vi "unescape string perf.vi"() -> ()   [LabVIEW 2017]
uses:
  JSONtext.lvlib
panel:
  in  "max length before escape":i32=10000000
  out "length after":i32
  out "length before":i32
  out "ds=":bool[](array[boolean])
  in  "unicode":bool=TRUE
  out "Array 2":string[](array[string])
  out "t":dbl[](array[numeric])=[1.4827295089180552, 2.8257225429488244, 2.876002117587632]
  # "lvjson"
  # "ds"
  # "lvjson"
  # "jsontxt"
  # "jsontxt"
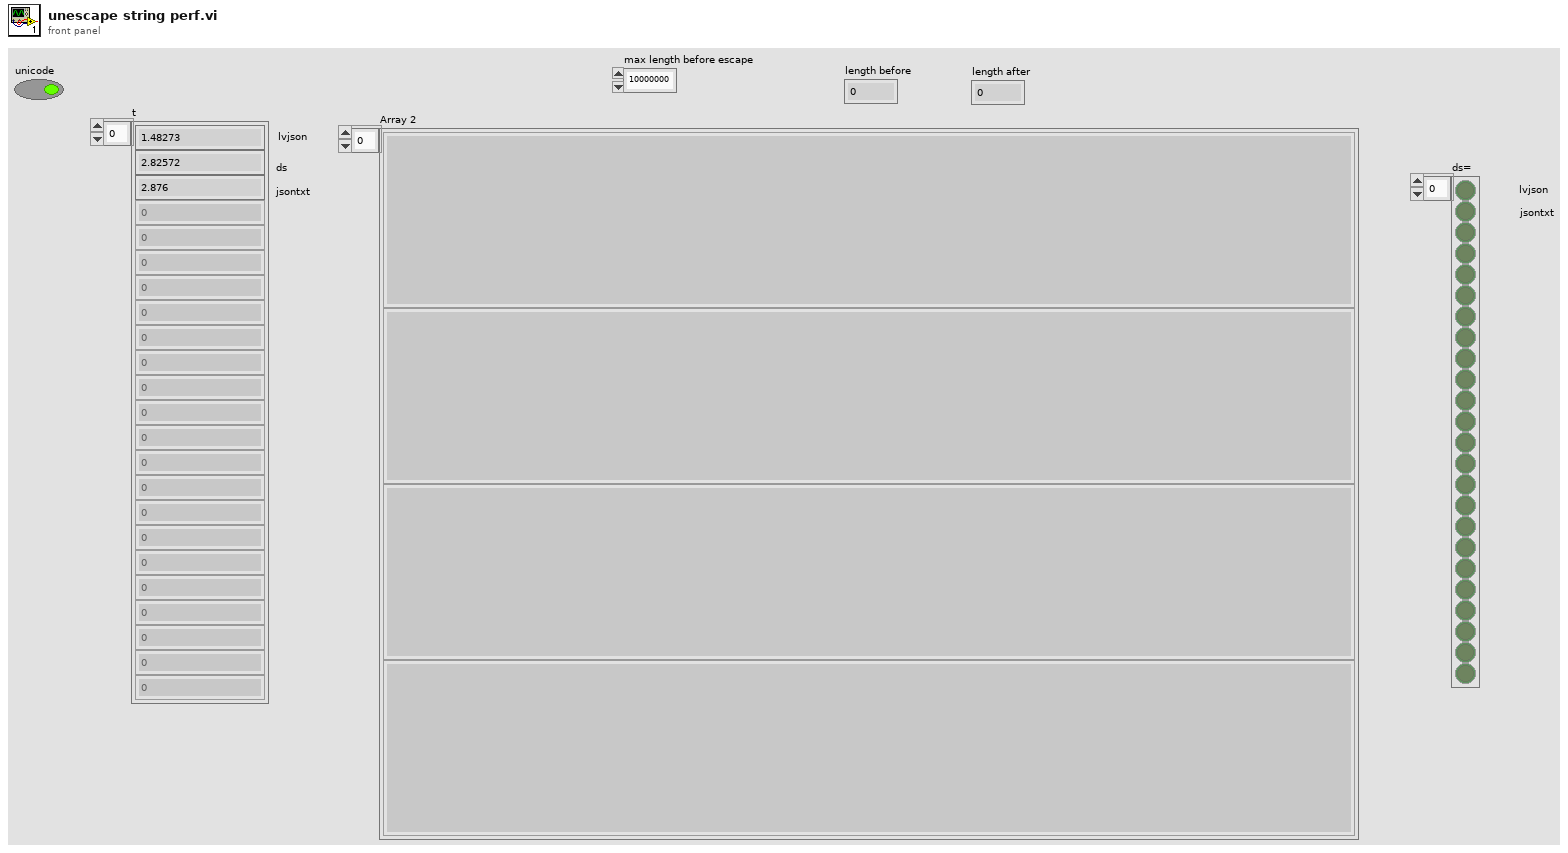
[diagram p1: front panel]
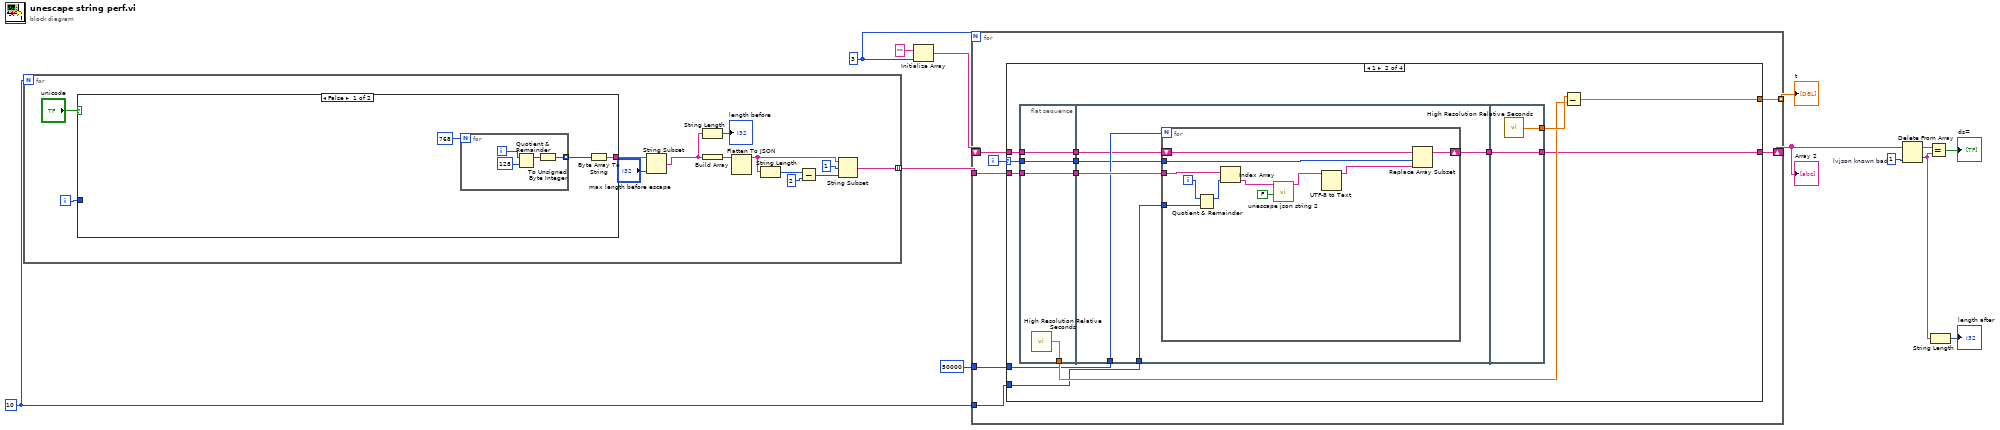
[diagram p0: block diagram]
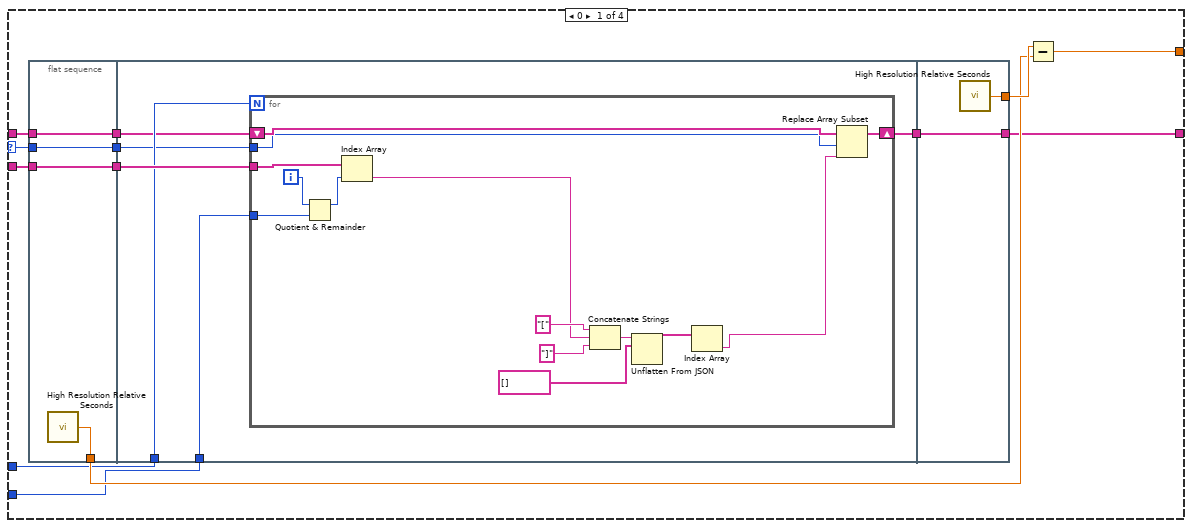
[diagram p2: hidden frame]
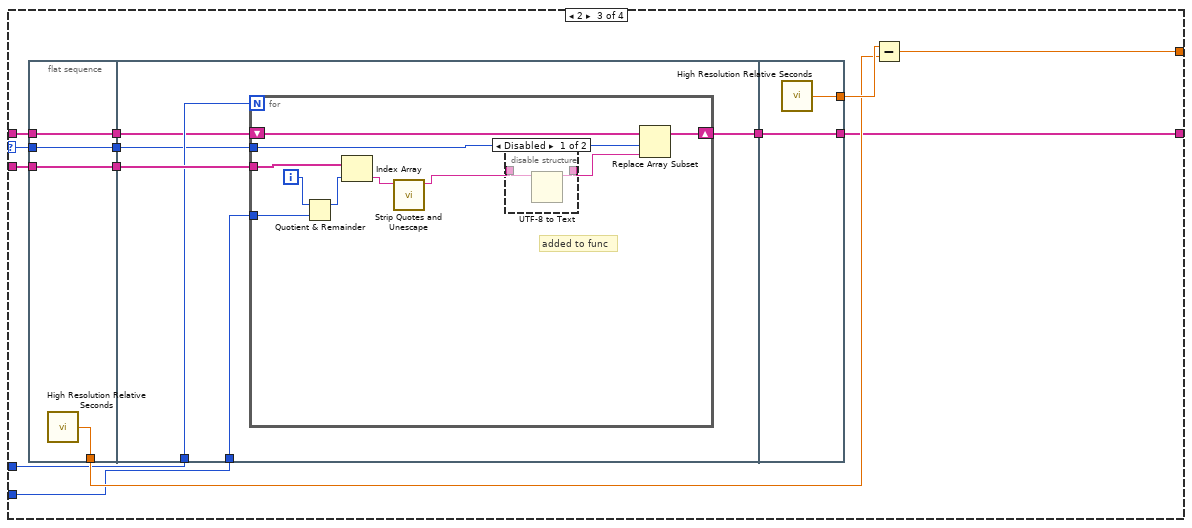
[diagram p3: hidden frame]
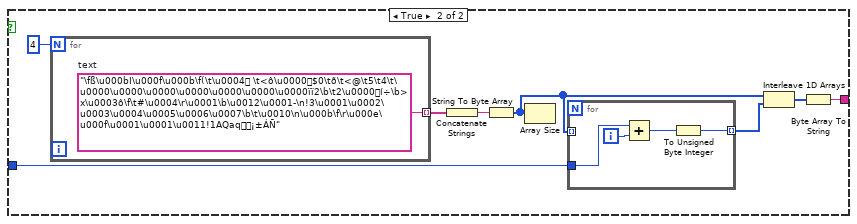
[diagram p6: hidden frame]
diagram:
  w4 = 1  # lvjson known bad
  w8 = 3
  w12 = 10
  n1 = for {
    N: w12 -> [_]
    tunnel: [w16] -> w10 mode=indexing
    i -> [w26]
    n2 = case shown="False" "unicode" {
      tunnel: w26 -> [_ w40]
      tunnel: [w27 w36] -> w17
      frame False {
        n3 = for {
          N: 768 -> [_]
          tunnel: [w30] -> w28 mode=indexing
          i -> [w33]
          n4 = Quotient & Remainder(x=w33, y=128) -> (x-y*floor(x/y)=w31:i32)  [unwired: 1 out]
          n5 = To Unsigned Byte Integer(number=w31) -> (unsigned 8bit integer=w30:u8)
        }
        n6 = Byte Array To String(unsigned byte array=w28) -> (string=w27:string)
      }
      frame True {
        n7 = for {
          N: 4 -> [_]
          tunnel: [w42] -> w41 mode=indexing
          w42 = "\fß\u000bI\u000f\u000b\f(\t\u0004 \t<ô\u0000$0\tð\t<@\t5\t4\t\u0000\u0000\u0000\u0000\u0000\u0000\u0000ïï2\b\t2\u0000í÷\b> x\u0003ô\f\t#\u0004\r\u0001\b\u0012\u0001-\n!3\u0001\u0002\u0003\u0004\u0005\u0006\u0007\b\t\u0010\n\u000b\f\r\u000e\u000f\u0001\u0001\u0011!1AQaq¡±ÁÑ"  # text
        }
        n8 = Concatenate Strings(w41) -> (w34:string)
        n9 = String To Byte Array(string=w34) -> (unsigned byte array=w38:u8[])
        n10 = Array Size(array=w38) -> ()  [unwired: 1 out]
        n11 = for {
          tunnel: w38 -> [_] mode=indexing
          tunnel: w40 -> [w45]
          tunnel: [w43] -> w39 mode=indexing
          i -> [w46]
          n12 = Add(x=w45, y=w46) -> (x+y=w44:i32)
          n13 = To Unsigned Byte Integer(number=w44) -> (unsigned 8bit integer=w43:u8)
        }
        n14 = Interleave 1D Arrays(w38, w39) -> (w37:u8[])
        n15 = Byte Array To String(unsigned byte array=w37) -> (string=w36:string)
      }
    }
    n16 = String Subset(string=w17, length (rest)="max length before escape") -> (substring=w15:string)  [unwired: 1 in]
    n17 = String Length(string=w15) -> (length=→"length before":i32)
    n18 = Build Array(w15) -> (w23:string[])
    n19 = Flatten To JSON(anything=w23) -> (JSON string=w21:string)  [unwired: 2 in, 1 out]
    n20 = String Length(string=w21) -> (length=w20:i32)
    n21 = Subtract(x=w20, y=2) -> (x-y=w18:i32)
    n22 = String Subset(string=w21, offset (0)=1, length (rest)=w18) -> (substring=w16:string)
  }
  n23 = Initialize Array("", w8) -> (w7:string[])
  n24 = for {
    N: w8 -> [_]
    tunnel: w10 -> [w51]
    tunnel: [w52] -> w13 mode=indexing
    tunnel: w12 -> [w50]
    tunnel: 50000 -> [w49]
    shift-right: [w47] -> w6
    shift-left: w7 -> [w48]
    i -> [w53]
    n25 = case shown="1" w53 {
      selector: w53 -> [w55 w94 w130 _]
      tunnel: [w64 w103 w139 _] -> w52
      tunnel: w51 -> [w62 w101 w137 _]
      tunnel: w50 -> [w61 w100 w136 _]
      tunnel: w49 -> [w60 w99 w135 _]
      tunnel: w48 -> [w59 w98 w134 w167]
      tunnel: [w57 w96 w132 w167] -> w47
      frame 0 {
        n26 = flat-sequence {
          tunnel: [w70] -> w65
          tunnel: [w69] -> w63
          tunnel: w62 -> [w69]
          tunnel: w59 -> [w68]
          tunnel: [w68] -> w58
          tunnel: w55 -> [w67]
          tunnel: [w67] -> w54
          tunnel: w63 -> [w75]
          tunnel: w61 -> [w76]
          tunnel: w60 -> [w74]
          tunnel: w58 -> [w73]
          tunnel: [w72] -> w56
          tunnel: w54 -> [w71]
          tunnel: [w92] -> w66
          tunnel: [w91] -> w57
          tunnel: w56 -> [w91]
          frame #0 {
            n27 = call <vilib>:"High Resolution Relative Seconds.vi"() -> ("relative seconds"=w70:dbl)
          }
          frame #1 {
            n28 = for {
              N: w74 -> [_]
              tunnel: w76 -> [w89]
              tunnel: w75 -> [w87]
              shift-right: [w85] -> w72
              shift-left: w73 -> [w86]
              tunnel: w71 -> [w84]
              i -> [w90]
              n29 = Quotient & Remainder(x=w90, y=w89) -> (x-y*floor(x/y)=w88:i32)  [unwired: 1 out]
              n30 = Index Array(array=w87, index=w88) -> (element=w78:string)
              n31 = Concatenate Strings("[", w78, "]") -> (w80:string)
              n32 = Unflatten From JSON(JSON string=w80, type and defaults=string[] []) -> (value=w79:string[])  [unwired: 5 in, 1 out]
              n33 = Index Array(array=w79) -> (element=w77:string)  [unwired: 1 in]
              n34 = Replace Array Subset(array=w86, new element=w77, index=w84) -> (w85:string[])
            }
          }
          frame #2 {
            n35 = call <vilib>:"High Resolution Relative Seconds.vi"() -> ("relative seconds"=w92:dbl)
          }
        }
        n36 = Subtract(x=w66, y=w65) -> (x-y=w64:dbl)
      }
      frame 1 {
        n37 = flat-sequence {
          tunnel: [w109] -> w104
          tunnel: [w108] -> w102
          tunnel: w101 -> [w108]
          tunnel: w98 -> [w107]
          tunnel: [w107] -> w97
          tunnel: w94 -> [w106]
          tunnel: [w106] -> w93
          tunnel: w102 -> [w114]
          tunnel: w100 -> [w115]
          tunnel: w99 -> [w113]
          tunnel: w97 -> [w112]
          tunnel: [w111] -> w95
          tunnel: w93 -> [w110]
          tunnel: [w128] -> w105
          tunnel: [w127] -> w96
          tunnel: w95 -> [w127]
          frame #0 {
            n38 = call <vilib>:"High Resolution Relative Seconds.vi"() -> ("relative seconds"=w109:dbl)
          }
          frame #1 {
            n39 = for {
              N: w113 -> [_]
              tunnel: w115 -> [w125]
              tunnel: w114 -> [w123]
              shift-right: [w121] -> w111
              shift-left: w112 -> [w122]
              tunnel: w110 -> [w120]
              i -> [w126]
              n40 = Quotient & Remainder(x=w126, y=w125) -> (x-y*floor(x/y)=w124:i32)  [unwired: 1 out]
              n41 = Index Array(array=w123, index=w124) -> (element=w118:string)
              n42 = call "unescape json string 2.vi"("quotes removed?"=FALSE, "base string"=w118) -> ("String out"=w116:string)  [unwired: 9 in]
              n43 = UTF-8 to Text(11:w116) -> (3:w119:string)  [unwired: 2 in, 1 out]
              n44 = Replace Array Subset(array=w122, new element=w119, index=w120) -> (w121:string[])
            }
          }
          frame #2 {
            n45 = call <vilib>:"High Resolution Relative Seconds.vi"() -> ("relative seconds"=w128:dbl)
          }
        }
        n46 = Subtract(x=w105, y=w104) -> (x-y=w103:dbl)
      }
      frame 2 {
        n47 = flat-sequence {
          tunnel: [w145] -> w140
          tunnel: [w144] -> w138
          tunnel: w137 -> [w144]
          tunnel: w134 -> [w143]
          tunnel: [w143] -> w133
          tunnel: w130 -> [w142]
          tunnel: [w142] -> w129
          tunnel: w138 -> [w150]
          tunnel: w136 -> [w151]
          tunnel: w135 -> [w149]
          tunnel: w133 -> [w148]
          tunnel: [w147] -> w131
          tunnel: w129 -> [w146]
          tunnel: [w166] -> w141
          tunnel: [w165] -> w132
          tunnel: w131 -> [w165]
          frame #0 {
            n48 = call <vilib>:"High Resolution Relative Seconds.vi"() -> ("relative seconds"=w145:dbl)
          }
          frame #1 {
            n49 = for {
              N: w149 -> [_]
              tunnel: w151 -> [w160]
              tunnel: w150 -> [w158]
              shift-right: [w156] -> w147
              shift-left: w148 -> [w157]
              tunnel: w146 -> [w155]
              i -> [w161]
              # "added to func"
              n50 = Quotient & Remainder(x=w161, y=w160) -> (x-y*floor(x/y)=w159:i32)  [unwired: 1 out]
              n51 = Index Array(array=w158, index=w159) -> (element=w154:string)
              n52 = call "Strip Quotes and Unescape.vi"("String"=w154) -> ("result string"=w153:string)  [unwired: 9 in, 1 out]
              n53 = disable-structure shown="Disabled" {
                disable-tunnel: w153 -> [w163 w164]
                disable-tunnel: [w162 w164] -> w152
                frame Disabled {
                  n54 = UTF-8 to Text(11:w163) -> (3:w162:string)  [unwired: 2 in, 1 out]
                }
                frame Enabled {
                }
              }
              n55 = Replace Array Subset(array=w157, new element=w152, index=w155) -> (w156:string[])
            }
          }
          frame #2 {
            n56 = call <vilib>:"High Resolution Relative Seconds.vi"() -> ("relative seconds"=w166:dbl)
          }
        }
        n57 = Subtract(x=w141, y=w140) -> (x-y=w139:dbl)
      }
      frame Default {
      }
    }
  }
  "t" <- w13
  "Array 2" <- w6
  n58 = Delete From Array(array=w6, index=w4) -> (deleted portion=w1:string, array with subset deleted=w3:string[])  [unwired: 1 in]
  n59 = Equal?(x=w3, y=w1) -> (x = y?=→"ds=":bool[])
  n60 = String Length(string=w1) -> (length=→"length after":i32)
